vi "calibrationElectrometer_getEvent_SettingsAppliedReadingSettings.vi"(8 "error in (no error)":errorcluster, 11 "logevent_SettingsApplied_ReadingSettings_Ctl":T1) -> (0 "error out":errorcluster, 2 "function return":i32, 3 "logevent_SettingsApplied_ReadingSettings_Ctl out":T1)   [LabVIEW 2016, in "SALLV_calibrationElectrometer.lvlib"]
doc: "int calibrationElectrometer_shm_getEvent_SettingsApplied_ReadingSettingsLV(calibrationElectrometer_logevent_SettingsApplied_ReadingSettingsLV *logevent_SettingsApplied_ReadingSettings_Ctl );"
uses:
  SALLV_calibrationElectrometer.lvlib
  DataTypes/logevent_SettingsApplied_ReadingSettings.ctl
  SALLV_calibrationElectrometer.so
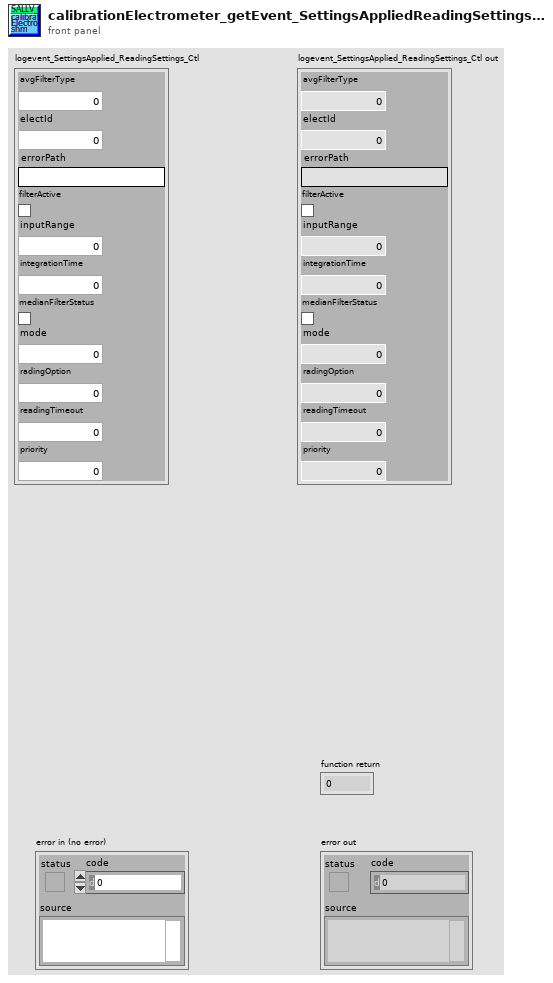
[diagram p1: front panel]
types:
  T1 = typedef "SALLV_calibrationElectrometer.lvlib/logevent_SettingsApplied_ReadingSettings.ctl" = cluster{"avgFilterType":i32, "electId":i16, "errorPath":string, "filterActive":bool, "inputRange":dbl, "integrationTime":dbl, "medianFilterStatus":bool, "mode":i32, "radingOption":i32, "readingTimeout":i32, "priority":i32}
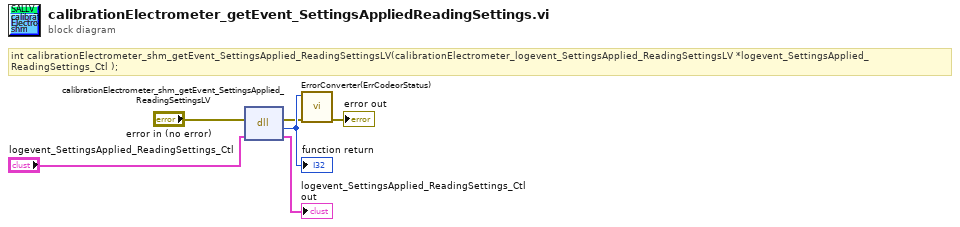
[diagram p0: block diagram]
diagram:
  # "int calibrationElectrometer_shm_getEvent_SettingsApplied_ReadingSettingsLV(calibrationElectrometer_logevent_SettingsApplied_ReadingSettingsLV *logevent_SettingsApplied_ReadingSettings_Ctl );"
  n1 = dll-call lib="home/andres/Desktop/SALLV_calibrationElectrometer/SALLV_calibrationElectrometer.*" fn="calibrationElectrometer_shm_getEvent_SettingsApplied_ReadingSettingsLV"(error in="error in (no error)", "logevent_SettingsApplied_ReadingSettings_Ctl"="logevent_SettingsApplied_ReadingSettings_Ctl") -> (error out=w2:errorcluster, w6:i32, "logevent_SettingsApplied_ReadingSettings_Ctl"=→"logevent_SettingsApplied_ReadingSettings_Ctl out":T1)  [unwired: 2 in, 1 out]
  "function return" <- w6
  n2 = call "ErrorConverter(ErrCodeorStatus).vi"("error in (no error)"=w2, "error code"=w6) -> ("error out"=→"error out":errorcluster)  [unwired: 9 in]
